vi "Ex2 Geometric Transformation.vi"() -> ()   [LabVIEW 2024]
panel:
  out "error out":errorcluster
  out "Image":T1(plugin-control)
  in  "Image Type":T2 items=["Grayscale (U8)", "Grayscale (I16)", "Grayscale (SGL)", "Complex (CSG)", "RGB (U32)", "HSL (U32)", "RGB (U64)", "Grayscale (U16)"]
  in  "File Path":path
  # "EX.2 GEOMETRIC TRANSFORMATION"
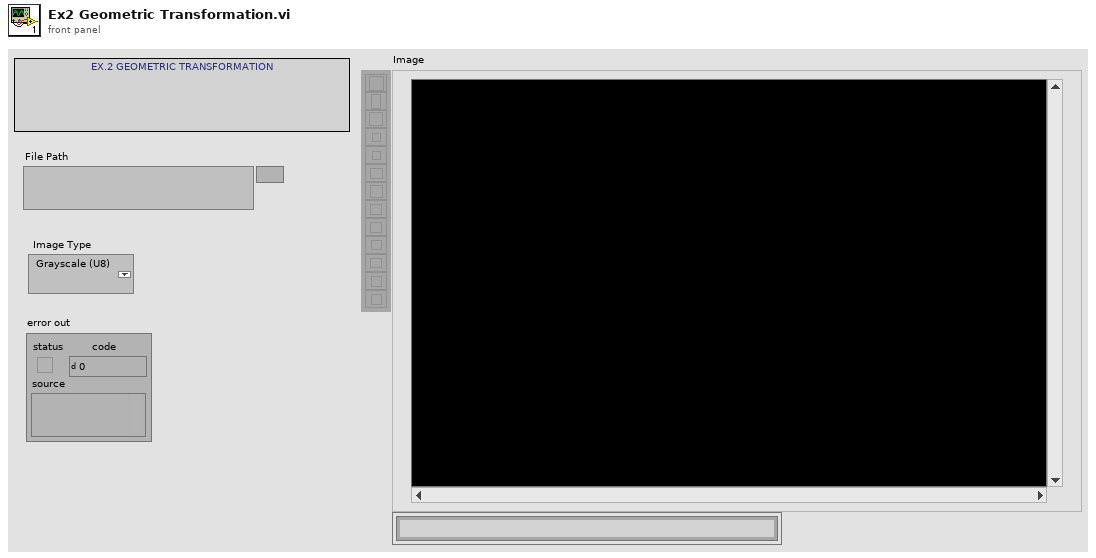
[diagram p1: front panel]
types:
  T1 = typedef "IMAQ Image.ctl" = refnum<image>
  T2 = typedef "Image Type" = u32
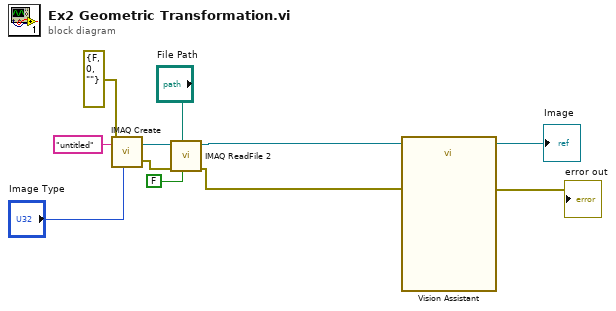
[diagram p0: block diagram]
diagram:
  n1 = call "IMAQ Create"("Image Name"="untitled", "Image Type"="Image Type", "error in (no error)"=errorcluster {"status"=FALSE, "code"=0, "source"=""}) -> ("New Image"=w7:T1, "error out"=w6:errorcluster)  [unwired: 2 in]
  n2 = call "IMAQ ReadFile 2"("Use File Path Image Type"=FALSE, "File Path"="File Path", "error in (no error)"=w6, "Image"=w7) -> ("error out"=w2:errorcluster, "Image Out"=w10:T1)  [unwired: 3 in, 3 out]
  n3 = call "Vision Assistant"("Image In"=w10, "error in"=w2) -> ("Image Out"=→"Image":T1, "error out"=→"error out":errorcluster)  [unwired: 24 in]
